vi "Finalize.vi"(8 "error in":errorcluster, 11 "Plugin in":refnum<class "Sift Stream.lvclass">) -> (0 "error out":errorcluster, 3 "Plugin out":refnum<class "Sift Stream.lvclass">)   [LabVIEW 2024, in "Sift Stream.lvlib" / "Sift Stream.lvclass"]
uses:
  Sift Stream.lvclass
  Sift Stream.lvclass/Sift Stream.ctl
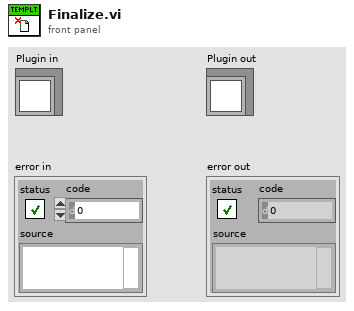
[diagram p1: front panel]
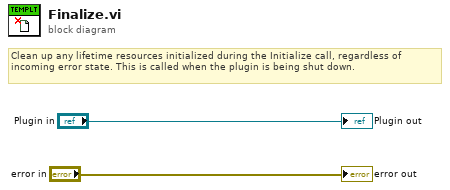
[diagram p0: block diagram]
diagram:
  # "Clean up any lifetime resources initialized during the Initialize call, regardless of incoming error state. This is called when the plugin is being shut down."
  "error out" <- "error in"
  "Plugin out" <- "Plugin in"
